vi "Robot Main.vi"() -> ()   [LabVIEW 2020]
doc: "This VI implements the framework and scheduler for your robotics program. It should not be necessary to modify the framework. You are expected to add your code to the VIs called from Robot Main - the ones located in the Team Code folder within the project."
uses:
  GlobalDriverStationData.vi
panel:
  in  "Finish":bool
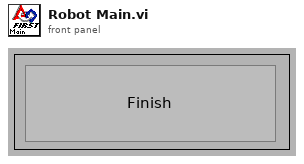
[diagram p1: front panel]
types:
  T1 = typedef "WPI_DriverStationMatch Info.ctl" = cluster{"Autonomous Elapsed Seconds":dbl, "TeleOp Elapsed Seconds":dbl, "Disabled Elapsed Seconds":dbl, "Visited Autonomous":bool, "Visited TeleOp":bool, "Visited Disabled":bool, "Autonomous Settings":cluster{"Autonomous Style":enum16{"Iterative", "Independent"}, "VI Refnum":refnum<vi>}}
  T2 = typedef "WPI_DriverStationDerivedRobotMode.ctl" = enum16{"Init", "Execute", "Stop"}
  T3 = typedef "WPI_DriverStationRobotMode2.ctl" = enum16{"Autonomous Disabled", "Autonomous Enabled", "Teleop Disabled", "Teleop Enabled", "Disconnected", "Finish", "Test Disabled", "Test Enabled", "Emergency Stopped"}
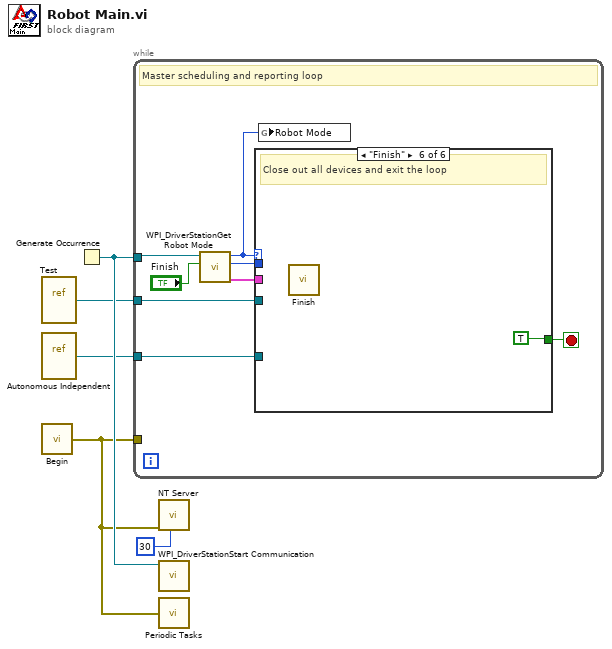
[diagram p0: block diagram]
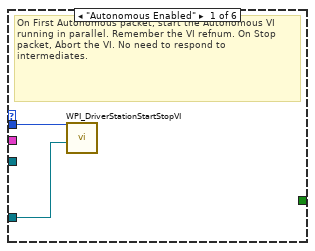
[diagram p2: hidden frame]
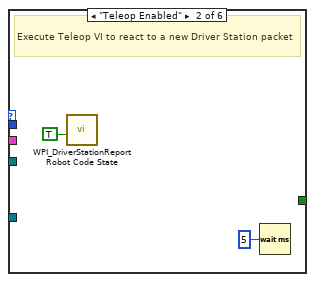
[diagram p3: hidden frame]
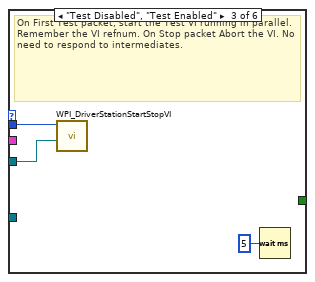
[diagram p4: hidden frame]
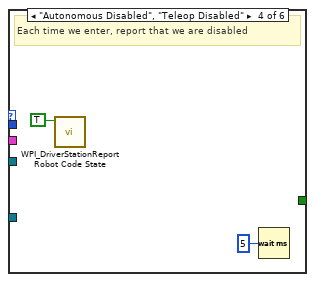
[diagram p5: hidden frame]
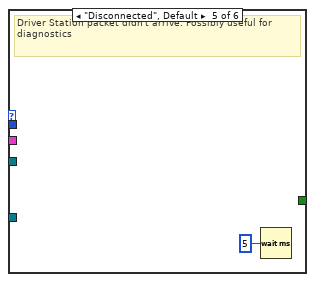
[diagram p6: hidden frame]
diagram:
  n1 = vi-ref "Test.vi"() -> (w3:refnum<vi>)
  n2 = vi-ref "Autonomous Independent.vi"() -> (w4:refnum<vi>)
  n3 = call "Begin.vi"() -> ("Error Out"=w2:errorcluster)  [unwired: 1 in]
  n4 = Generate Occurrence() -> (w5:refnum<k4>)
  n5 = while "Scheduling loop" {
    tunnel: w5 -> [w12]
    tunnel: w2 -> [_]
    tunnel: w4 -> [w8]
    tunnel: w3 -> [w7]
    stop <- w9 stop-if-true
    # "Master scheduling and reporting loop"
    n6 = call <vilib>:"WPI_DriverStationGet Robot Mode.vi"("Finish"="Finish", "DS Occurrence"=w12) -> ("Match Info out"=w10:T1, "Call Context"=w13:T2, "Robot Mode"=w6:T3)  [unwired: 7 out]
    n7 = case shown="\"Finish\"" w6 {
      tunnel: w13 -> [w15 _ w20 _ _ _]
      tunnel: w10 -> [_ _ _ _ _ _]
      tunnel: [_ _ _ _ _ TRUE] -> w9
      tunnel: w8 -> [w14 _ _ _ _ _]
      tunnel: w7 -> [_ _ w19 _ _ _]
      frame "Autonomous Enabled" {
        # "On First Autonomous packet, start the Autonomous VI running in parallel. Remember the VI refnum. On Stop packet, Abort the VI. No need to respond to intermediates."
        n8 = call <vilib>:"WPI_DriverStationStartStopVI.vi"("VI in"=w14, "Call Context"=w15) -> ()  [unwired: 10 in]
      }
      frame "Teleop Enabled" {
        # "Execute Teleop VI to react to a new Driver Station packet"
        n9 = call <vilib>:"WPI_DriverStationReport Robot Code State.vi"("TeleOp"=TRUE ("Autonomous")) -> ()  [unwired: 10 in, 1 out]
        n10 = Wait (ms)(milliseconds to wait=u32 5) -> ()  [unwired: 1 out]
      }
      frame "Test Disabled", "Test Enabled" {
        # "On First Test packet, start the Test VI running in parallel. Remember the VI refnum. On Stop packet Abort the VI. No need to respond to intermediates."
        n11 = call <vilib>:"WPI_DriverStationStartStopVI.vi"("VI in"=w19, "Call Context"=w20) -> ()  [unwired: 10 in]
        n12 = Wait (ms)(milliseconds to wait=u32 5) -> ()  [unwired: 1 out]
      }
      frame "Autonomous Disabled", "Teleop Disabled" {
        # "Each time we enter, report that we are disabled"
        n13 = call <vilib>:"WPI_DriverStationReport Robot Code State.vi"("Disabled"=TRUE ("Autonomous")) -> ()  [unwired: 10 in, 1 out]
        n14 = Wait (ms)(milliseconds to wait=u32 5) -> ()  [unwired: 1 out]
      }
      frame "Disconnected", Default {
        # "Driver Station packet didn't arrive. Possibly useful for diagnostics"
        n15 = Wait (ms)(milliseconds to wait=u32 5) -> ()  [unwired: 1 out]
      }
      frame "Finish" {
        # "Close out all devices and exit the loop"
        n16 = call "Finish.vi"() -> ()  [unwired: 1 in]
      }
    }
    n17 = global write "GlobalDriverStationData.vi" "Robot Mode"(w6) -> ()
  }
  n18 = call <vilib>:"NT Server.vi"("Update Time"=30, "error in (no error)"=w2) -> ()  [unwired: 9 in, 1 out]
  n19 = call <vilib>:"WPI_DriverStationStart Communication.vi"("occurrence"=w5) -> ()  [unwired: 2 in, 9 out]
  n20 = call "Periodic Tasks.vi"("error in"=w2) -> ()
